vi "Configure NetworkStream Server.vi"(6 "timeout (500 ms)":i32=500, 8 "error in (no error)":errorcluster, 9 "Stream Name":string="StreamName", 10 "Context":string="serverContext") -> (0 "error out":errorcluster, 3 "Connection.NetworkStream":refnum<class "Connection.NetworkStream.lvclass">)   [LabVIEW 2013, in "Connection.NetworkQueue_GOSPL.lvlib" / "Connection.NetworkStream.lvclass"]
uses:
  Connection.NetworkStream/Connection.NetworkStream.lvclass
  Connection/Connection.lvclass/Connection.ctl
  Connection/Connection.lvclass
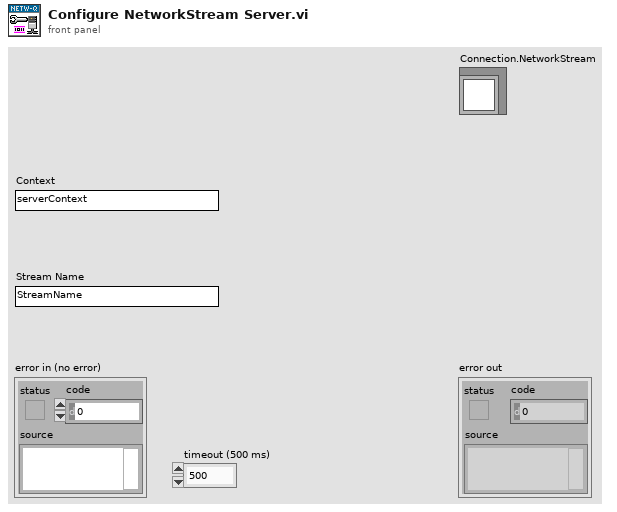
[diagram p1: front panel]
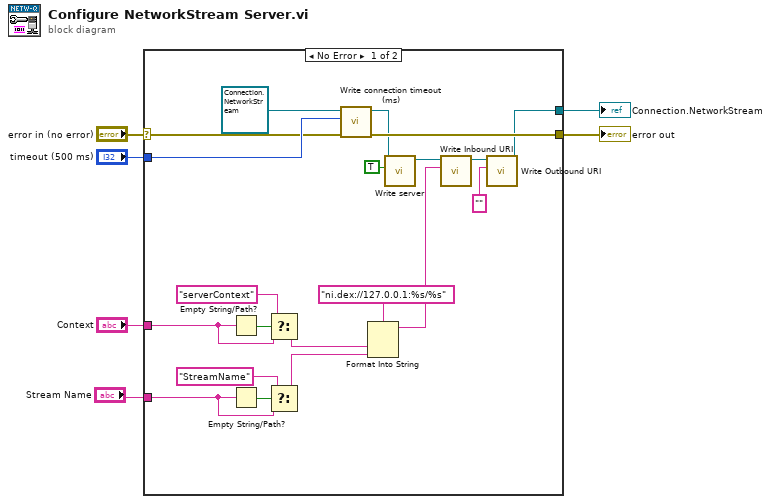
[diagram p0: block diagram]
diagram:
  n1 = case shown="No Error" "error in (no error)" {
    selector: "error in (no error)" -> [w25 w27]
    tunnel: [w24 w27] -> w5
    tunnel: [w11 _] -> w3
    tunnel: "timeout (500 ms)" -> [w26 _]
    tunnel: "Context" -> [w21 _]
    tunnel: "Stream Name" -> [w18 _]
    frame No Error {
      n2 = Empty String/Path?(string/path=w21) -> (empty?=w22:bool)
      n3 = Empty String/Path?(string/path=w18) -> (empty?=w19:bool)
      n4 = Select(t="serverContext", s=w22, f=w21) -> (s? t:f=w16:string)
      n5 = Select(t="StreamName", s=w19, f=w18) -> (s? t:f=w17:string)
      n6 = call "Write connection timeout (ms).vi"("error in (no error)"=w25, "connection timeout (ms)"=w26, "Connection in"=refnum<class "Connection.NetworkStream.lvclass"> refnum ("Connection.LocalQueue")) -> ("error out"=w24:errorcluster, "Connection out"=w9:refnum<class "Connection.NetworkStream.lvclass">)  [unwired: 7 in]
      n7 = Format Into String(format string="ni.dex://127.0.0.1:%s/%s", w16, w17) -> (resulting string=w13:string)  [unwired: 2 in, 1 out]
      n8 = call "Write server.vi"("server"=TRUE, "Connection in"=w9) -> ("Connection out"=w7:refnum<class "Connection.NetworkStream.lvclass">)  [unwired: 9 in]
      n9 = call "Write Inbound URI.vi"("Inbound URI"=w13, "Connection in"=w7) -> ("Connection out"=w12:refnum<class "Connection.NetworkStream.lvclass">)  [unwired: 9 in]
      n10 = call "Write Outbound URI.vi"("Outbound URI"="" ("Outbound Stream URI"), "Connection in"=w12) -> ("Connection out"=w11:refnum<class "Connection.NetworkStream.lvclass">)  [unwired: 9 in]
    }
    frame Error {
    }
  }
  "error out" <- w5
  "Connection.NetworkStream" <- w3
